vi "SEA_9811_Start.vi"(8 "error in (no error)":errorcluster, 11 "SEA9811_RT_data in":T1) -> (0 "error out":errorcluster, 3 "SEA9811_RT_data out":T1)   [LabVIEW 2012]
uses:
  Typdefs/SEA9811_RT_data_cluster.ctl
  <userlib>/_FPGA Interface Advanced Tools/FPGA Interface Base/FPGA Interface Base.lvclass
  Typdefs/FPGA ref.ctl
  Typdefs/channel.ctl
  Typdefs/received word.ctl
  Typdefs/SEA9811_FPGA_FP_Addresses.ctl
  <userlib>/_FPGA Interface Advanced Tools/FPGA Interface Base/FPGA Write By Name - Boolean.vi
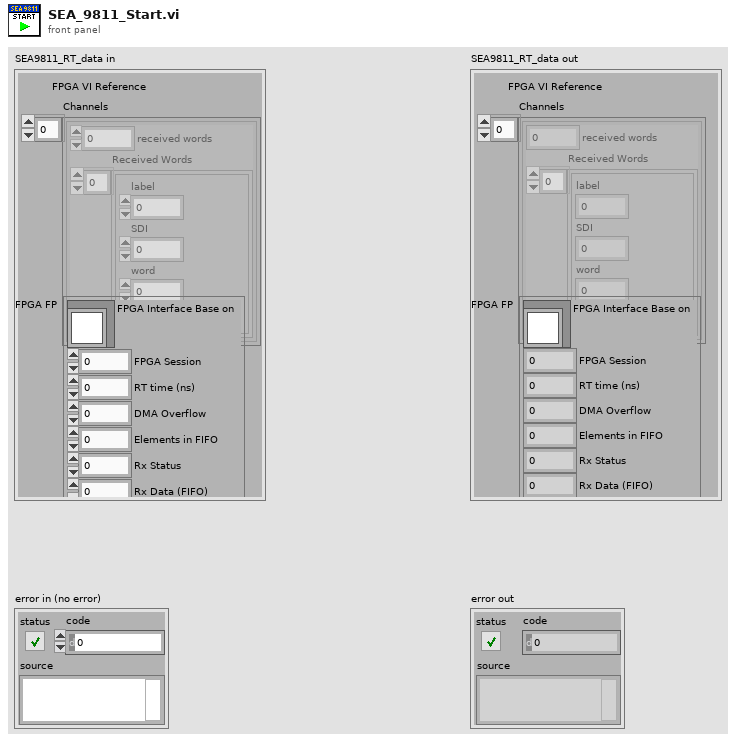
[diagram p1: front panel]
types:
  T1 = typedef "SEA9811_RT_data_cluster.ctl" = cluster{"FPGA VI Reference":T2, "Channels":T3[], "FPGA FP":T5}
  T2 = typedef "FPGA ref.ctl" = refnum<k20>
  T3 = typedef "channel.ctl" = cluster{"received words":u32, "Received Words":T4[]}
  T4 = typedef "received word.ctl" = cluster{"label":u8, "SDI":u8, "word":u32, "timestamp":dbl}
  T5 = typedef "SEA9811_FPGA_FP_Addresses.ctl" = cluster{"FPGA Interface Base on":refnum<class "FPGA Interface Base.lvclass">, "FPGA Session":u32, "RT time (ns)":u32, "DMA Overflow":u32, "Elements in FIFO":u32, "Rx Status":u32, "Rx Data (FIFO)":u32}
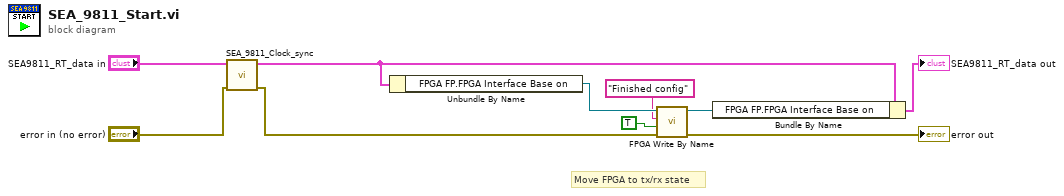
[diagram p0: block diagram]
diagram:
  # "Move FPGA to tx/rx state"
  n1 = call "SEA_9811_Clock_sync.vi"("error in (no error)"="error in (no error)", "SEA9811_RT_data in"="SEA9811_RT_data in") -> ("error out"=w1:errorcluster, "SEA9811_RT_data out"=w3:T1)  [unwired: 8 in]
  n2 = Unbundle By Name(w3) -> ("FPGA FP.FPGA Interface Base on"=w9:refnum<class "FPGA Interface Base.lvclass">)
  n3 = call-poly <userlib>:"FPGA Write By Name.vi"("error in (no error)"=w1, "Value"=TRUE ("Finished config"), "Control"="Finished config", "FPGA Session In"=w9) -> ("error out"=→"error out":errorcluster, "FPGA Session Out"=w6:refnum<class "FPGA Interface Base.lvclass">)  [unwired: 6 in]
  n4 = Bundle By Name(cluster=w3, "FPGA FP.FPGA Interface Base on"=w6) -> (→"SEA9811_RT_data out":T1)
